vi "Initialize with Switch Parameters Core.vi"(8 "error in (no error)":errorcluster, 10 "Switch Parameters in":refnum<class "Abstract Switch Init Parameters.lvclass">, 11 "Test Switch Consumer in":refnum<class "Test Switch Consumer.lvclass">) -> (0 "error out":errorcluster, 3 "Test Switch Consumer out":refnum<class "Test Switch Consumer.lvclass">)   [LabVIEW 2017, in "Test Switch Consumer.lvclass"]
uses:
  Test Switch Consumer.lvclass
  Switch/Abstract Switch Init Parameters/Abstract Switch Init Parameters.lvclass
  Test Switch Init Parameters/Test Switch Init Parameters.lvclass
  Test Switch Init Parameters/Test Switch Init Parameters.lvclass/Test Switch Init Parameters.ctl
  Test Switch Consumer.lvclass/Test Switch Consumer.ctl
  Test Switch Init Parameters/Read Test Param.vi
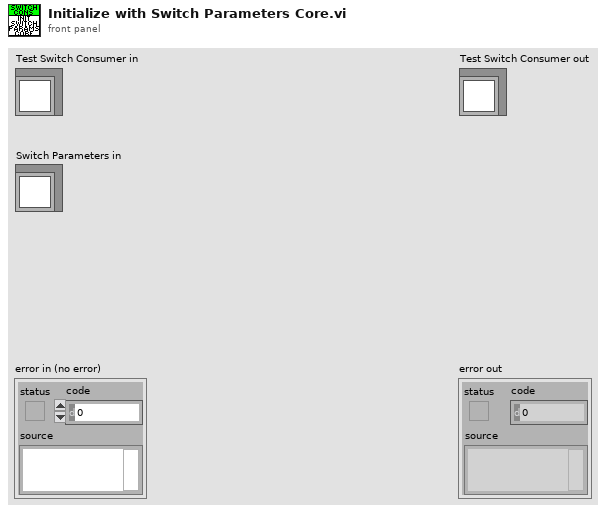
[diagram p1: front panel]
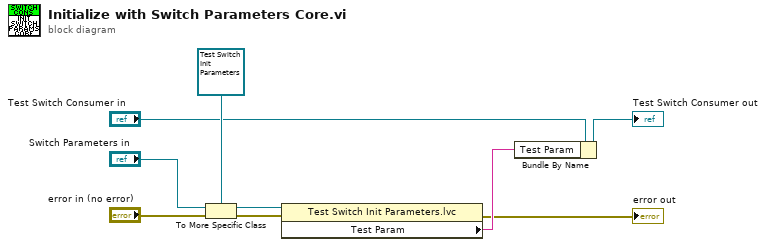
[diagram p0: block diagram]
diagram:
  n1 = To More Specific Class(target class=refnum<class "Test Switch Init Parameters.lvclass"> refnum ("Test Switch Init Parameters.lvclass"), reference="Switch Parameters in", error in="error in (no error)") -> (specific class reference=w6:refnum<class "Test Switch Init Parameters.lvclass">, error out=w5:errorcluster)
  n2 = property class="Test Switch Init Parameters.lvc"(reference=w6, error in=w5) -> (error out=→"error out":errorcluster, "Test Param"=w3:string)  [unwired: 1 out]
  n3 = Bundle By Name(cluster="Test Switch Consumer in", "Test Param"=w3) -> (→"Test Switch Consumer out":refnum<class "Test Switch Consumer.lvclass">)
